vi "Setting.vi"(8 "error constant":errorcluster, 11 "DAQ Config":T1) -> (0 "error out":errorcluster, 2 "Canceled":bool, 3 "DAQ Config out":T1)   [LabVIEW 2017]
uses:
  Control/Config chanel.ctl
  <vilib>/Utility/xml.llb/Write to XML File(string).vi
panel:
  in  "Cancel Button":bool
  in  "OK Button":bool
  in  "Minimum Input":dbl=-10.0
  in  "Maximum Input":dbl=10.0
  in  "Samples Read":dbl
  in  "DAQmx Channel":tag
  in  "Sampling Rate":dbl
  in  "Log File Path":path
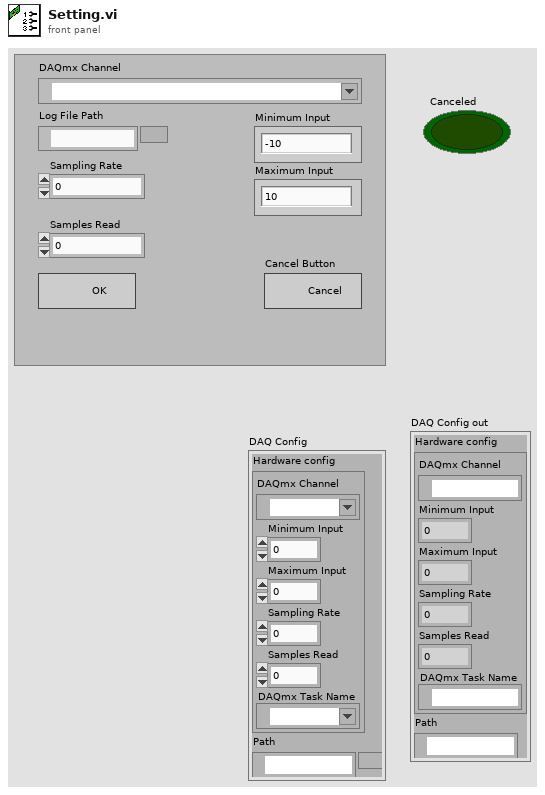
[diagram p1: front panel]
types:
  T1 = typedef "Config chanel.ctl" = cluster{"Hardware config":cluster{"DAQmx Channel":tag, "Minimum Input":dbl, "Maximum Input":dbl, "Sampling Rate":dbl, "Samples Read":dbl, "DAQmx Task Name":refnum<k21>}, "Path":path}
  T2 = typedef "Config chanel.ctl" = cluster{"Path":path, "DAQmx Channel":tag, "Minimum Input":dbl, "Maximum Input":dbl, "Sampling Rate":dbl, "Samples Read":dbl, "DAQmx Task Name":refnum<k21>}
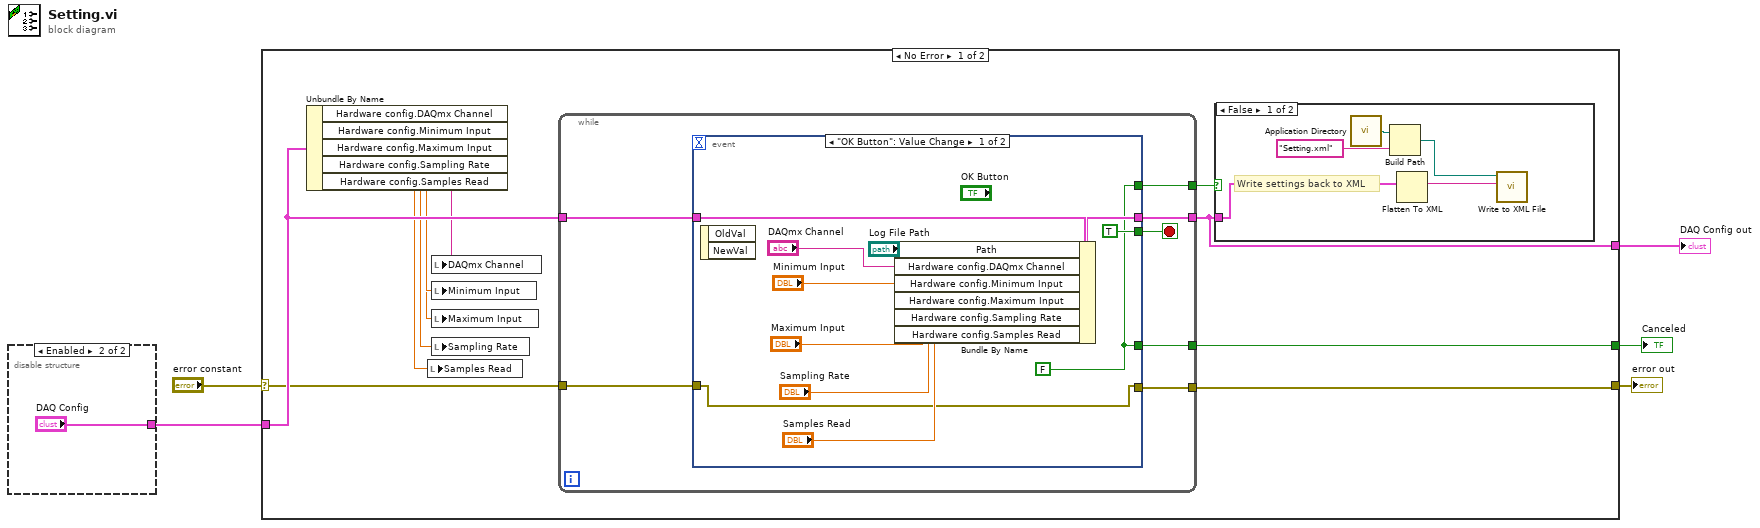
[diagram p0: block diagram]
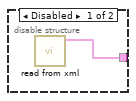
[diagram p2: hidden frame]
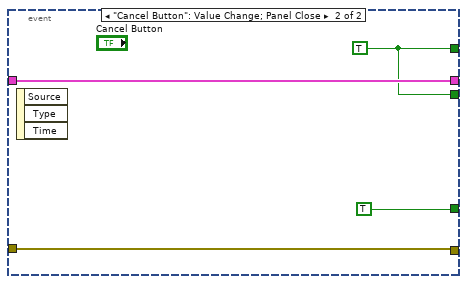
[diagram p4: hidden frame]
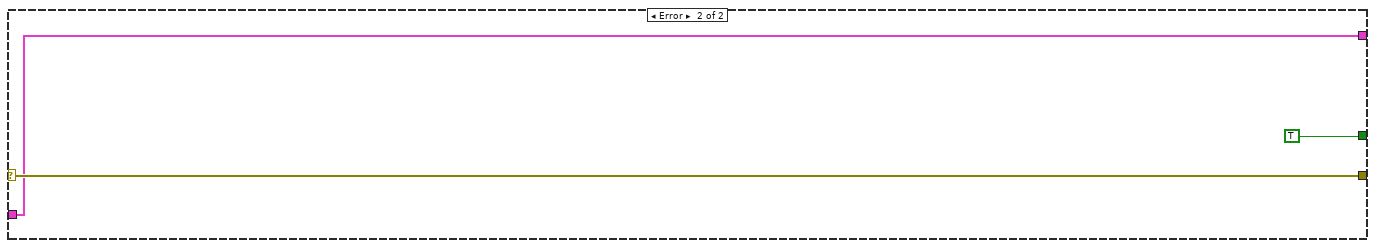
[diagram p5: hidden frame]
diagram:
  n1 = disable-structure shown="Enabled" {
    disable-tunnel: [w6 "DAQ Config"] -> w2
    frame Disabled {
      n2 = call "read from xml.vi"() -> ("DAQ Config"=w6:T2)  [unwired: 10 in, 1 out]
    }
    frame Enabled {
    }
  }
  n3 = case shown="No Error" "error constant" {
    selector: "error constant" -> [w10 w48]
    tunnel: w2 -> [w18 w47]
    tunnel: [w12 w47] -> w3
    tunnel: [w9 w48] -> w4
    tunnel: [w8 TRUE] -> w1
    frame No Error {
      n4 = Unbundle By Name(w18) -> ("Hardware config.DAQmx Channel"=w17:tag, "Hardware config.Minimum Input"=w16:dbl, "Hardware config.Maximum Input"=w15:dbl, "Hardware config.Sampling Rate"=w14:dbl, "Hardware config.Samples Read"=w11:dbl)
      n5 = local write "Samples Read"(w11) -> ()
      n6 = local write "DAQmx Channel"(w17) -> ()
      n7 = local write "Minimum Input"(w16) -> ()
      n8 = local write "Maximum Input"(w15) -> ()
      n9 = local write "Sampling Rate"(w14) -> ()
      n10 = while {
        tunnel: w18 -> [w30]
        tunnel: [w29] -> w12
        tunnel: [w27] -> w13
        tunnel: w10 -> [w26]
        tunnel: [w25] -> w9
        tunnel: [w24] -> w8
        stop <- w28 stop-if-true
        n11 = event shown="[0] \"OK Button\": Value Change" {
          selector: _ -> [_ _]
          dyn-events: _ -> [_ _]
          timeout: _ -> [_ _]
          tunnel: w30 -> [w41 w44]
          tunnel: [w32 w44] -> w29
          tunnel: [TRUE w43] -> w28
          tunnel: [w31 w43] -> w27
          tunnel: [w33 w45] -> w25
          tunnel: w26 -> [w33 w45]
          tunnel: [w31 TRUE] -> w24
          event "OK Button": Value Change {
            w31 = FALSE
            n12 = event-data() -> ()  [unwired: 1 in, 2 out]
            n13 = Bundle By Name(cluster=w41, "Path"="Log File Path", "Hardware config.DAQmx Channel"="DAQmx Channel", "Hardware config.Minimum Input"="Minimum Input", "Hardware config.Maximum Input"="Maximum Input", "Hardware config.Sampling Rate"="Sampling Rate", "Hardware config.Samples Read"="Samples Read") -> (w32:T1)
          }
          event "Cancel Button": Value Change; Panel Close {
            w43 = TRUE
            n14 = event-data() -> ()  [unwired: 1 in, 3 out]
          }
        }
      }
      n15 = case shown="False" w13 {
        tunnel: w12 -> [w23 _]
        frame False {
          # "Write settings back to XML"
          n16 = call <vilib>:"Application Directory.vi"() -> ("Application Directory"=w22:path)
          n17 = Build Path(base path=w22, name or relative path="Setting.xml") -> (appended path=w20:path)
          n18 = Flatten To XML(anything=w23) -> (xml string=w19:string)
          n19 = call-poly <vilib>:"Write to XML File.vi"("XML Input"=w19, "XML File Path"=w20) -> ()  [unwired: 7 in, 3 out]
        }
        frame True {
        }
      }
    }
    frame Error {
    }
  }
  "error out" <- w4
  "DAQ Config out" <- w3
  "Canceled" <- w1
